vi "xio.listdir_lua.vi"(5 "LuaVIEW reference":T1) -> (15 "error out":errorcluster)   [LabVIEW 2012]
doc: "Lists the content of a directory or a VI library. The listed files and/or directories are returned as full paths.\n\nTo get a recursive listing, bind the \"Library Recursively List Files.vi\" in the library/file handling/ directory or simply use the following function:\n<pre><code>function xio.recursedir(path)\n local files,dirs=xio.listdir(path)\n for i,d in ipairs(dirs) do\n for j,f in ipairs(xio.recursedir(d)) do\n table.insert(files,f)\n end\n end\n return files\nend</code></pre>\nParameters:\nstr:path, directory or llb to list.\n[str:pattern], filter pattern that can use the ? and * wildcards.\nResults:\ntab:files, paths of the files in the directory or llb being listed.\ntab:dirs, paths of the subdirectories of the directory being listed.\nErrors:\nNot a directory.\nNo such directory.\nAccess denied."
uses:
  typedefs/t_LuaVIEW Reference.ctl
  subvis/private/LuaVIEW Pull (path).vi
  subvis/private/LuaVIEW Pull (string).vi
  subvis/private/LuaVIEW Push (flat data).vi
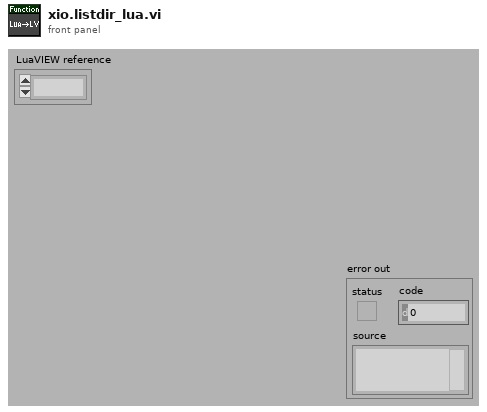
[diagram p1: front panel]
types:
  T1 = typedef "t_LuaVIEW Reference.ctl" = refnum<k1>
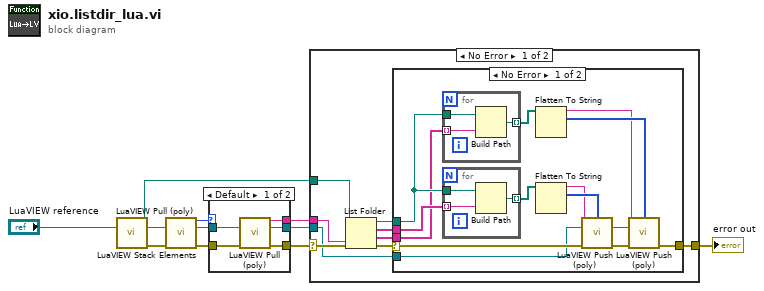
[diagram p0: block diagram]
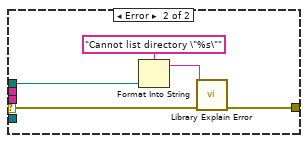
[diagram p3: hidden frame]
diagram:
  n1 = call-poly "LuaVIEW Pull (poly).vi"("LuaVIEW reference in"="LuaVIEW reference") -> ("path"=w11:path, "LuaVIEW reference out"=w7:T1, "error out"=w8:errorcluster)  [unwired: 12 in]
  n2 = call "LuaVIEW Stack Elements.vi"("LuaVIEW reference in"=w7, "error in (no error)"=w8) -> ("elements"=w6:i32, "LuaVIEW reference out"=w4:T1, "error out"=w5:errorcluster)  [unwired: 11 in]
  n3 = case shown="Default" w6 {
    tunnel: w5 -> [w16 w18]
    tunnel: w4 -> [w15 w17]
    tunnel: [w14 _] -> w3
    tunnel: [w13 w18] -> w2
    tunnel: [w12 w17] -> w1
    frame Default {
      n4 = call-poly "LuaVIEW Pull (poly).vi"("LuaVIEW reference in"=w15, "error in (no error)"=w16) -> ("string"=w14:string, "LuaVIEW reference out"=w12:T1, "error out"=w13:errorcluster)  [unwired: 11 in]
    }
    frame 0 {
    }
  }
  n5 = case shown="No Error" w2 {
    selector: w2 -> [w27 w53]
    tunnel: w11 -> [w20 _]
    tunnel: [w25 w53] -> w10
    tunnel: w3 -> [w23 _]
    tunnel: w1 -> [w19 _]
    frame No Error {
      n6 = List Folder(path=w20, pattern=w23, error in=w27) -> (path out=w21:path, filenames=w24:string[], folder names=w22:string[], error out=w26:errorcluster)  [unwired: 1 in]
      n7 = case shown="No Error" w26 {
        selector: w26 -> [w41 w52]
        tunnel: [w35 w51] -> w25
        tunnel: w24 -> [w33 _]
        tunnel: w22 -> [w32 _]
        tunnel: w21 -> [w38 w48]
        tunnel: w19 -> [w40 _]
        frame No Error {
          n8 = for {
            tunnel: w38 -> [w47]
            tunnel: w32 -> [w46] mode=indexing
            tunnel: [w45] -> w39 mode=indexing
            n9 = Build Path(base path=w47, name or relative path=w46) -> (appended path=w45:path)
          }
          n10 = for {
            tunnel: w38 -> [w44]
            tunnel: w33 -> [w43] mode=indexing
            tunnel: [w42] -> w34 mode=indexing
            n11 = Build Path(base path=w44, name or relative path=w43) -> (appended path=w42:path)
          }
          n12 = Flatten To String(anything=w39) -> (data string=w30:string, type string=w31:i16[])  [unwired: 3 in, 1 out]
          n13 = Flatten To String(anything=w34) -> (data string=w28:string, type string=w29:i16[])  [unwired: 3 in, 1 out]
          n14 = call-poly "LuaVIEW Push (poly).vi"("flat data"=w28, "type descriptor"=w29, "LuaVIEW reference in"=w40, "error in (no error)"=w41) -> ("LuaVIEW reference out"=w36:T1, "error out"=w37:errorcluster)  [unwired: 10 in]
          n15 = call-poly "LuaVIEW Push (poly).vi"("flat data"=w30, "type descriptor"=w31, "LuaVIEW reference in"=w36, "error in (no error)"=w37) -> ("error out"=w35:errorcluster)  [unwired: 10 in, 1 out]
        }
        frame Error {
          n16 = Format Into String(format string="Cannot list directory \"%s\"", w48) -> (resulting string=w50:string)  [unwired: 2 in, 1 out]
          n17 = call "Library Explain Error.vi"("explanation prefix (none)"=w50, "error in (no error)"=w52) -> ("explained error"=w51:errorcluster)  [unwired: 13 in]
        }
      }
    }
    frame Error {
    }
  }
  "error out" <- w10
